vi "Read_Write_INI.vi"(0 "Process_Data_In":T1[][](array[typedef]), 5 "File_Path":path, 11 "Error_In":errorcluster, 13 "INI_Select":T2) -> (4 "Process_Data_Out":T1[][](array[typedef]), 15 "Error_Out":errorcluster)   [LabVIEW 2023]
doc: "Used to read and write the INI file."
uses:
  Control/INI_Operation_Select.ctl
  Control/Stage_Data.ctl
  <vilib>/Utility/config.llb/Read Key (String).vi
  <vilib>/Utility/config.llb/NI_LVConfig.lvlib
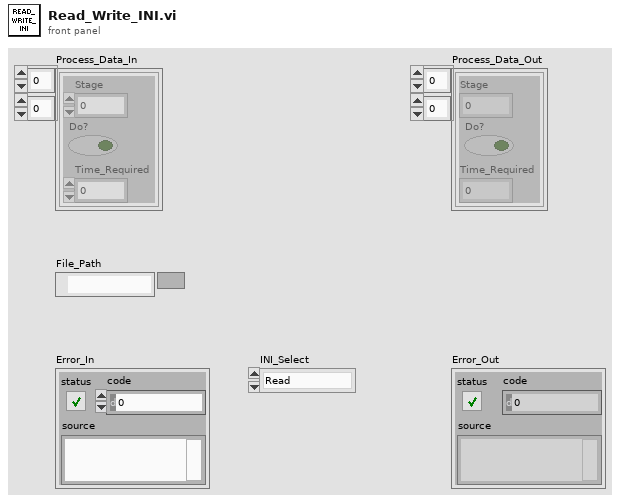
[diagram p1: front panel]
types:
  T1 = typedef "Stage_Data.ctl" = cluster{"Stage":i32, "Do?":bool, "Time_Required":i32}
  T2 = typedef "INI_Operation_Select.ctl" = enum16{"Read", "Write"}
  T3 = typedef "NI_LVConfig.lvlib/Config Data RefNum.ctl" = refnum<k1>
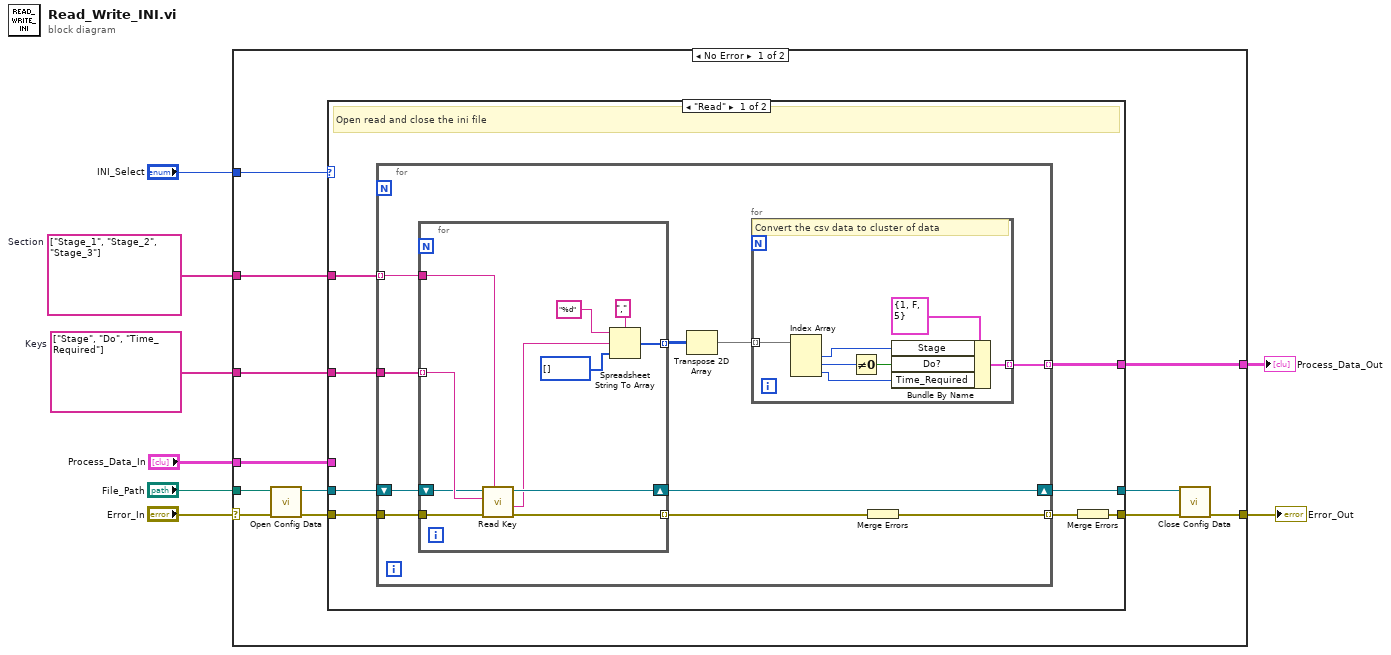
[diagram p0: block diagram]
diagram:
  w4 = string[] ["Stage_1", "Stage_2", "Stage_3"]  # Section
  w5 = string[] ["Stage", "Do", "Time_Required"]  # Keys
  n1 = case shown="No Error" "Error_In" {
    selector: "Error_In" -> [w16 w59]
    tunnel: [w20 w59] -> w8
    tunnel: "File_Path" -> [w19 _]
    tunnel: "INI_Select" -> [w18 _]
    tunnel: w5 -> [w17 _]
    tunnel: w4 -> [w11 _]
    tunnel: [w10 _] -> w3
    tunnel: "Process_Data_In" -> [w9 _]
    frame No Error {
      n2 = call <vilib>:"Open Config Data.vi"("error in (no error)"=w16, "configuration file path"=w19) -> ("error out"=w15:errorcluster, "refnum"=w14:T3)  [unwired: 7 in, 1 out]
      n3 = case shown="\"Read\"" w18 {
        tunnel: w15 -> [w27 w58]
        tunnel: [w23 w58] -> w13
        tunnel: w17 -> [w28 _]
        tunnel: w14 -> [w26 w57]
        tunnel: [w25 w57] -> w12
        tunnel: w11 -> [w22 _]
        tunnel: [w21 _] -> w10
        tunnel: w9 -> [_ _]
        frame "Read" {
          # "Open read and close the ini file"
          n4 = for {
            tunnel: w28 -> [w38]
            tunnel: w27 -> [w37]
            tunnel: [w32] -> w24 mode=indexing
            tunnel: w22 -> [w33] mode=indexing
            tunnel: [w29] -> w21 mode=indexing
            shift-right: [w35] -> w25
            shift-left: w26 -> [w36]
            n5 = for {
              tunnel: w38 -> [w56] mode=indexing
              tunnel: w33 -> [w51]
              shift-right: [w53] -> w35
              shift-left: w36 -> [w54]
              tunnel: w37 -> [w55]
              tunnel: [w52] -> w34 mode=indexing
              tunnel: [w47] -> w31 mode=indexing
              n6 = call-poly <vilib>:"Read Key.vi"("section"=w51, "error in (no error)"=w55, "key"=w56, "refnum"=w54) -> ("error out"=w52:errorcluster, "value"=w50:string, "refnum out"=w53:T3)  [unwired: 4 in, 1 out]
              n7 = Spreadsheet String To Array(delimiter (Tab)=",", format string="%d", spreadsheet string=w50, array type (2D Dbl)=i32[] []) -> (array=w47:i32[])
            }
            n8 = Transpose 2D Array(2D array=w31) -> (transposed array=w30:i32[][])
            n9 = for {
              tunnel: [w40] -> w29 mode=indexing
              tunnel: w30 -> [w39] mode=indexing
              # "Convert the csv data to cluster of data"
              n10 = Index Array(array=w39) -> (element #1=w44:i32, element #2=w42:i32, element #3=w43:i32)  [unwired: 3 in]
              n11 = Not Equal To 0?(x=w42) -> (x != 0?=w41:bool)
              n12 = Bundle By Name(cluster=T1 {"Stage"=1, "Do?"=FALSE, "Time_Required"=5} ("Process_Details"), "Stage"=w44, "Do?"=w41, "Time_Required"=w43) -> (w40:T1)
            }
            n13 = Merge Errors(w34) -> (w32:errorcluster)
          }
          n14 = Merge Errors(w24) -> (w23:errorcluster)
        }
        frame "Write" {
          # "#TODO \nWriting is not needed for this assignment but added for future implementation"
          # "Open write and close the ini file"
        }
      }
      n15 = call <vilib>:"Close Config Data.vi"("error in (no error)"=w13, "refnum"=w12) -> ("error out"=w20:errorcluster)  [unwired: 8 in, 1 out]
    }
    frame Error {
    }
  }
  "Error_Out" <- w8
  "Process_Data_Out" <- w3
